vi "bufferPosition1.vi"(3 "Input String":string) -> (0 "Output 21":string, 1 "Output 22":string, 2 "Output 23":string, 4 "Output 24":string, 5 "Output 27":string, 6 "Output 25":string, 7 "Output 26":string, 8 "Output 16":string, 9 "Output 20":string, 10 "Output 15":string, 11 "Output 19":string, 12 "Output 14":string, 13 "Output 18":string, 14 "Output 13":string, 15 "Output 17":string, 16 "Output 12":string, 17 "Output1":string, 18 "Output 11":string, 19 "Output 2":string, 20 "Output 10":string, 21 "Output 9":string, 22 "Output 8":string, 23 "Output 7":string, 24 "Output 6":string, 25 "Output 5":string, 26 "Output 4":string, 27 "Output 3":string)   [LabVIEW 2015]
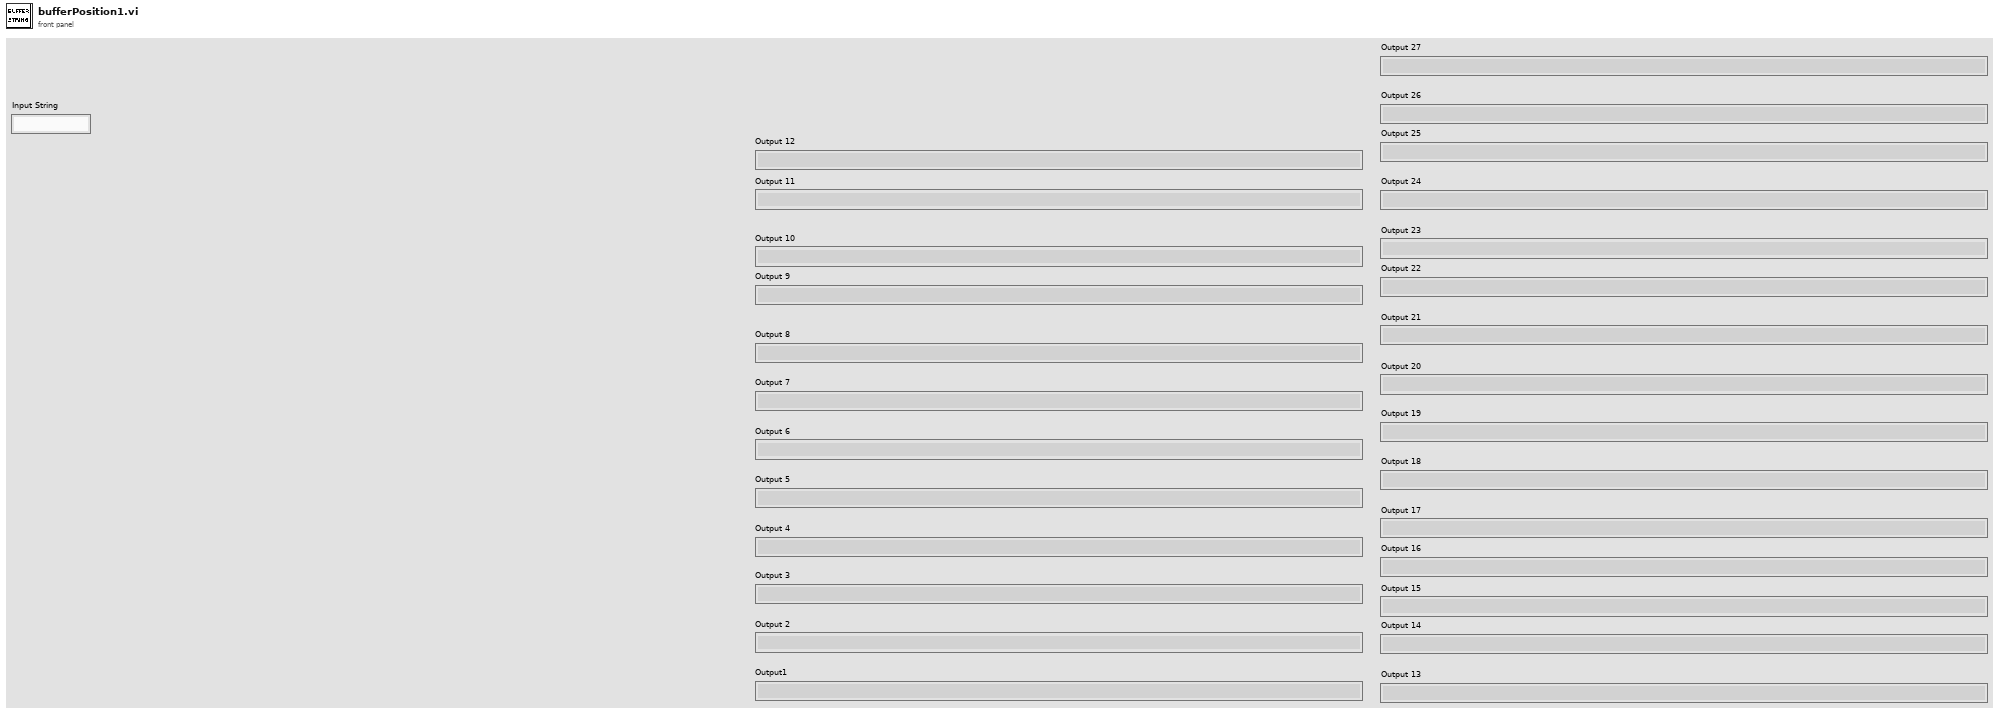
[diagram p1: front panel]
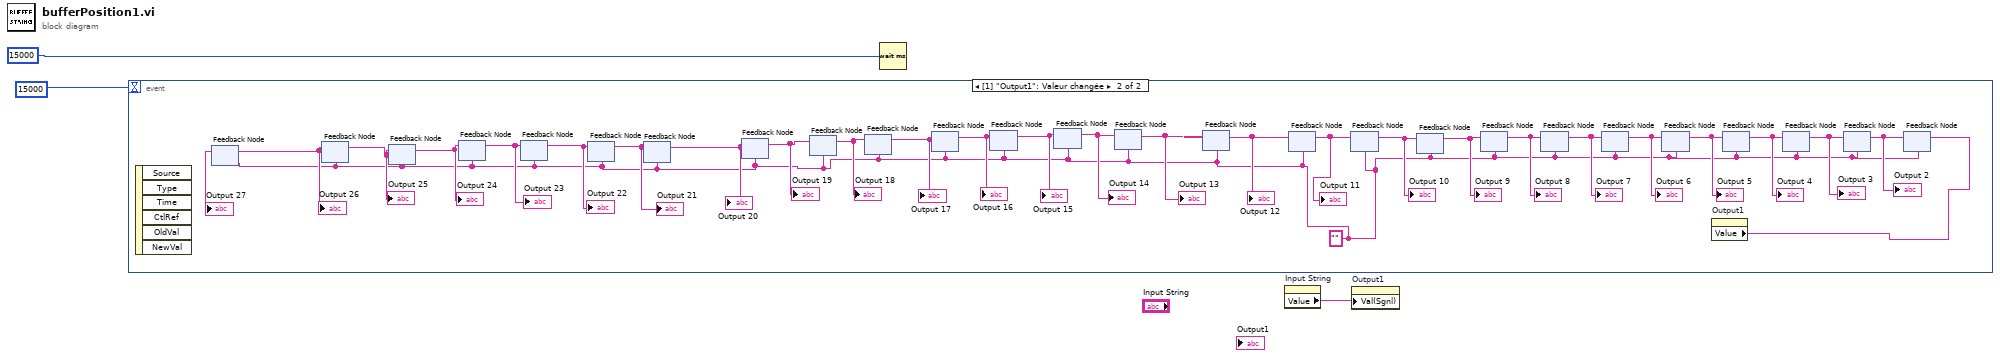
[diagram p0: block diagram]
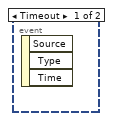
[diagram p2: hidden frame]
diagram:
  n1 = event shown="[1] \"Output1\": Valeur changée" {
    selector: _ -> [_ _]
    dyn-events: _ -> [_ _]
    timeout: 15000 -> [_ _]
    event Timeout {
      n2 = event-data() -> ()  [unwired: 1 in, 3 out]
    }
    event "Output1": Value Change {
      w5 = ""
      n3 = event-data() -> ()  [unwired: 1 in, 6 out]
      n4 = feedback #1(w5) -> (→"Output 27":string)
      n5 = feedback #2(w5) -> (w6:string)
      "Output 26" <- w6
      n6 = feedback-in #1(w6) -> ()
      n7 = feedback #3(w5) -> (w7:string)
      "Output 25" <- w7
      n8 = feedback-in #2(w7) -> ()
      n9 = feedback #4(w5) -> (w8:string)
      "Output 24" <- w8
      n10 = feedback-in #3(w8) -> ()
      n11 = feedback #5(w5) -> (w9:string)
      "Output 23" <- w9
      n12 = feedback-in #4(w9) -> ()
      n13 = feedback #6(w5) -> (w10:string)
      "Output 22" <- w10
      n14 = feedback-in #5(w10) -> ()
      n15 = feedback #7(w5) -> (w11:string)
      "Output 21" <- w11
      n16 = feedback-in #6(w11) -> ()
      n17 = feedback #8(w5) -> (w12:string)
      "Output 20" <- w12
      n18 = feedback-in #7(w12) -> ()
      n19 = feedback #9(w5) -> (w13:string)
      "Output 19" <- w13
      n20 = feedback-in #8(w13) -> ()
      n21 = feedback #10(w5) -> (w14:string)
      "Output 18" <- w14
      n22 = feedback-in #9(w14) -> ()
      n23 = feedback #11(w5) -> (w15:string)
      "Output 17" <- w15
      n24 = feedback-in #10(w15) -> ()
      n25 = feedback #12(w5) -> (w16:string)
      "Output 16" <- w16
      n26 = feedback-in #11(w16) -> ()
      n27 = feedback #13(w5) -> (w17:string)
      "Output 15" <- w17
      n28 = feedback-in #12(w17) -> ()
      n29 = feedback #14(w5) -> (w18:string)
      "Output 14" <- w18
      n30 = feedback-in #13(w18) -> ()
      n31 = feedback #15(w5) -> (w19:string)
      "Output 13" <- w19
      n32 = feedback-in #14(w19) -> ()
      n33 = feedback #16(w5) -> (w20:string)
      "Output 12" <- w20
      n34 = feedback-in #15(w20) -> ()
      n35 = feedback #17(w5) -> (w22:string)
      "Output 11" <- w22
      n36 = feedback-in #16(w22) -> ()
      n37 = feedback #18(w5) -> (w25:string)
      "Output 10" <- w25
      n38 = feedback-in #17(w25) -> ()
      n39 = feedback #19(w5) -> (w26:string)
      "Output 9" <- w26
      n40 = feedback-in #18(w26) -> ()
      n41 = feedback #20(w5) -> (w27:string)
      "Output 8" <- w27
      n42 = feedback-in #19(w27) -> ()
      n43 = feedback #21(w5) -> (w28:string)
      "Output 7" <- w28
      n44 = feedback-in #20(w28) -> ()
      n45 = feedback #22(w5) -> (w29:string)
      "Output 6" <- w29
      n46 = feedback-in #21(w29) -> ()
      n47 = property on="Output1" class="Ch"() -> ("Value"=w21:string)  [unwired: 2 in, 2 out]
      n48 = feedback #23(w5) -> (w30:string)
      "Output 5" <- w30
      n49 = feedback-in #22(w30) -> ()
      n50 = feedback #24(w5) -> (w31:string)
      "Output 4" <- w31
      n51 = feedback-in #23(w31) -> ()
      n52 = feedback #25(w5) -> (w23:string)
      "Output 3" <- w23
      n53 = feedback-in #24(w23) -> ()
      n54 = feedback #26(w5) -> (w24:string)
      "Output 2" <- w24
      n55 = feedback-in #25(w24) -> ()
      n56 = feedback-in #26(w21) -> ()
    }
  }
  n57 = Wait (ms)(milliseconds to wait=u32 15000) -> ()  [unwired: 1 out]
  n58 = property on="Input String" class="Ch"() -> ("Value"=w1:string)  [unwired: 2 in, 2 out]
  n59 = property on="Output1" class="Ch"("Val(Sgnl)"=w1) -> ()  [unwired: 2 in, 2 out]
